vi "Configure Serial Bus Type.vi"(8 "error in (no error)":errorcluster, 9 "Serial Bus Type (0: CAN)":i32(ring) items=["CAN", "I2S", "IIC", "LIN", "SPI", "UART", "A429", "FlexRay", "M1553", "SENT", "CXPI", "Manchester", "NRZ", "USB PD", "USB"], 10 "Serial Bus Name (1: Serial Bus 1)":i32(ring)=1 items=["Serial Bus 1"=1, "Serial Bus 2"=2], 11 "VISA resource name":refnum<visa-resource-name>) -> (0 "error out":errorcluster, 3 "VISA resource name out":refnum<visa-resource-name>)   [LabVIEW 2017, in "Agilent 2000 3000 X-Series.lvlib"]
doc: "Configures serial bus type."
uses:
  Agilent 2000 3000 X-Series.lvlib
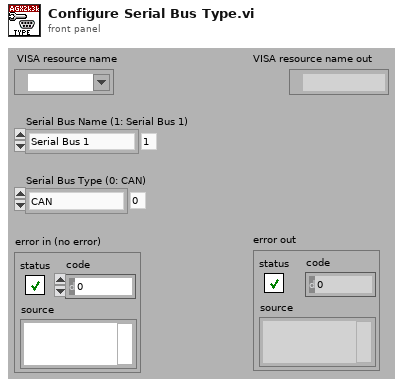
[diagram p1: front panel]
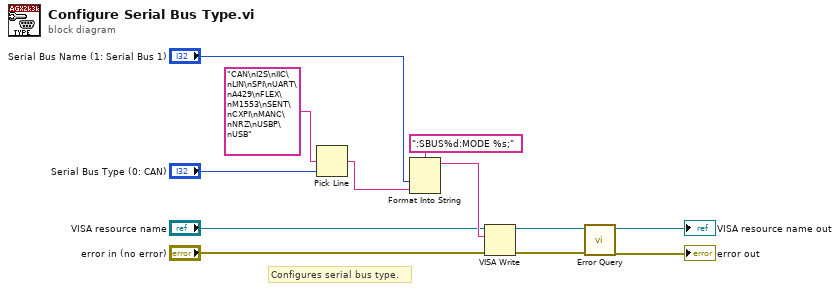
[diagram p0: block diagram]
diagram:
  # "Configures serial bus type."
  n1 = Pick Line(multi-line string="CAN\nI2S\nIIC\nLIN\nSPI\nUART\nA429\nFLEX\nM1553\nSENT\nCXPI\nMANC\nNRZ\nUSBP\nUSB", line index="Serial Bus Type (0: CAN)") -> (output string=w8:string)  [unwired: 1 out]
  n2 = Format Into String(format string=":SBUS%d:MODE %s;", "Serial Bus Name (1: Serial Bus 1)", w8) -> (resulting string=w7:string)  [unwired: 2 in, 1 out]
  n3 = VISA Write(VISA resource name="VISA resource name", write buffer=w7, error in (no error)="error in (no error)") -> (VISA resource name out=w4:refnum<visa-resource-name>, error out=w3:errorcluster)  [unwired: 1 out]
  n4 = call "Error Query.vi"("error in (no error)"=w3, "VISA resource name"=w4) -> ("error out"=→"error out":errorcluster, "VISA resource name out"=→"VISA resource name out":refnum<visa-resource-name>)  [unwired: 8 out]
